vi "Read Nested Libraries.vi"(8 "error in (no error)":errorcluster, 11 "Lib in":refnum<class "Lib.lvclass">) -> (0 "error out":errorcluster, 2 "Nested Libraries":T1[](array[typedef]), 3 "Lib out":refnum<class "Lib.lvclass">)   [LabVIEW 2021, in "TAF Proj Document Type.lvlib" / "Lib.lvclass"]
uses:
  <vilib>/Wovalab/AntiDoc/Document Type/Add-ons/LabVIEW TAF Project/Lib/Lib.lvclass
  <vilib>/Wovalab/AntiDoc/Document Type/Add-ons/LabVIEW TAF Project/Lib/Nested Lib Info--cluster.ctl
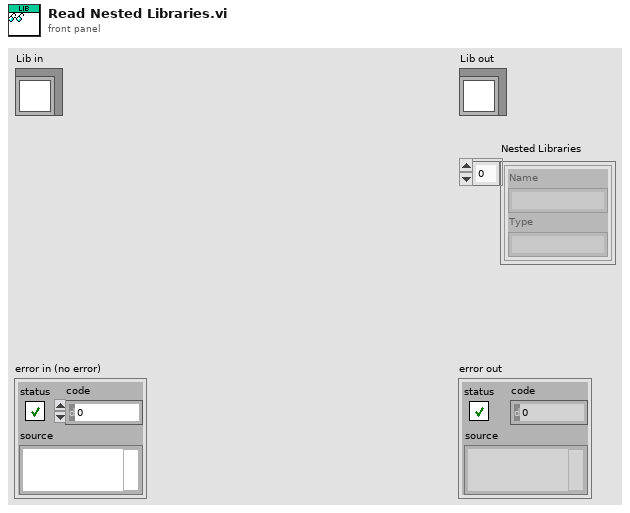
[diagram p1: front panel]
types:
  T1 = typedef "TAF Proj Document Type.lvlib/Lib.lvclass/Nested Lib Info--cluster.ctl" = cluster{"Name":string, "Type":string}
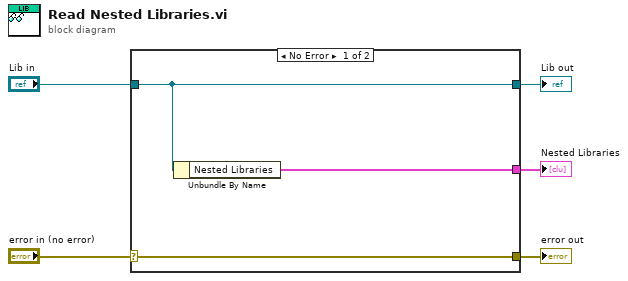
[diagram p0: block diagram]
diagram:
  n1 = case shown="No Error" "error in (no error)" {
    selector: "error in (no error)" -> [w8 w9]
    tunnel: [w8 w9] -> w4
    tunnel: [w7 w10] -> w2
    tunnel: "Lib in" -> [w7 w10]
    tunnel: [w6 _] -> w1
    frame No Error {
      n2 = Unbundle By Name(w7) -> ("Nested Libraries"=w6:T1[])
    }
    frame Error {
    }
  }
  "error out" <- w4
  "Lib out" <- w2
  "Nested Libraries" <- w1
